vi "PH_GetPowermeterInformation.PC Get Info.vi"(2 "MCL Listbox GUI Ref":refnum<vi>, 5 "error in":errorcluster) -> (19 "error out":errorcluster)   [LabVIEW 2014, in "PH_GetPowermeterInformation.lvlib"]
doc: "This is the proc case \"get information\"."
uses:
  PH_GetPowermeterInformation.lvlib
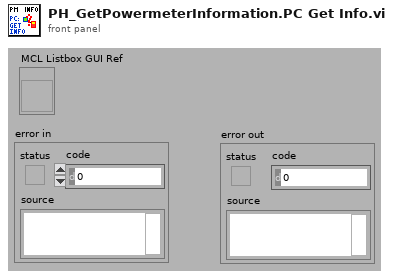
[diagram p1: front panel]
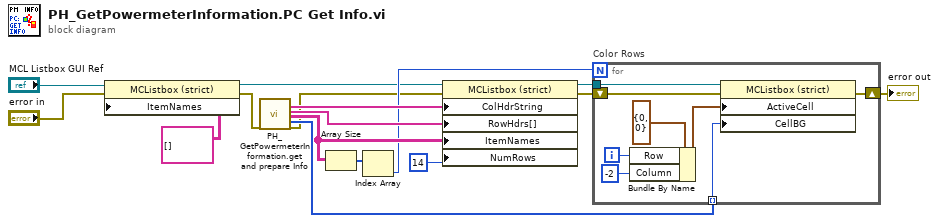
[diagram p0: block diagram]
diagram:
  n1 = property class="MCListbox (strict)"(reference="MCL Listbox GUI Ref", error in="error in", "ItemNames"=string[][] [] ("Item Names")) -> (reference out=w3:refnum<vi>, error out=w5:errorcluster)
  n2 = call "PH_GetPowermeterInformation.get and prepare Info.vi"("error in"=w5) -> ("ColHdrs[]"=w12:string[], "RowHdrs[]"=w11:string[], "ItemNames"=w13:string[][], "Row Cell BG"=w14:u32[], "error out"=w4:errorcluster)  [unwired: 14 in]
  n3 = Array Size(array=w13) -> (size(s)=w10:i32[])
  n4 = Index Array(array=w10) -> (element=w6:i32)  [unwired: 1 in]
  n5 = property class="MCListbox (strict)"(reference=w3, error in=w4, "ColHdrString"=w12, "RowHdrs[]"=w11, "ItemNames"=w13, "NumRows"=u32 14 ("Number of Rows")) -> (reference out=w7:refnum<vi>, error out=w8:errorcluster)
  n6 = for "Color Rows" {
    N: w6 -> [_]
    tunnel: w7 -> [w22]
    shift-right: [w23] -> w2
    shift-left: w8 -> [w24]
    tunnel: w14 -> [w19] mode=indexing
    i -> [w18]
    n7 = Bundle By Name(cluster=cluster{"Row":i32, "Column":i32} {"Row"=0, "Column"=0} ("Active Cell:Active Cell"), "Row"=w18, "Column"=-2 ("Row")) -> (w21:cluster{"Row":i32, "Column":i32})
    n8 = property class="MCListbox (strict)"(reference=w22, error in=w24, "ActiveCell"=w21, "CellBG"=w19) -> (error out=w23:errorcluster)  [unwired: 1 out]
  }
  "error out" <- w2
